vi "ScanBuilder.vi"(2 "Selected\nScan\nCorners":dbl[][](array[numeric])=[[211.0, 177.0, 58.0], [316.0, 213.0, 58.0]], 3 "ROI_Array 2":T3(array[cluster]) {"ROI begin channel" step=0.001; "ROI end channel" step=0.001; "Intensity" step=0.001; "Net Intensity" step=0.001; "Gauss Fit" step=0.001; "FWHM [keV]" step=0.001; "Center [keV]" step=0.001}) -> (0 "Do?":bool, 1 "ScanData":T4)   [LabVIEW 2015]
uses:
  Controls/String.ctl
  Controls/Number.ctl
panel:
  in  "PresetROI":u16(ring) items=["ca", "scat", "fe", "scat"]
  in  "Snake?":bool
  in  "Scan order:":u16(ring)=1 items=["X->Z->Y"=6, "Y->Z->X"=5, "Z->X->Y"=3, "Y->X->Z"=2, "Z->Y->X"=4, "X->Y->Z"=1]
  out "estimated duration":string caption="Estimated duration:"
  out "Output\nScan\nCorners":dbl[][](array[numeric])=[[211.0, 177.0, 58.0], [316.0, 213.0, 58.0]]
  in  "Accept":bool
  in  "Scan definition by:":enum32{"Step size", "Number of steps"}(radio)
  in  "Y steps":i32=1 min=1 step=1
  in  "X steps":i32=1 min=1 step=1
  out "total # of points":i32=1 min=0 step=1
  in  "step Y [mm]":dbl=1.0 min=0.0 step=0.1
  in  "step X [mm]":dbl=1.0 min=0.0 step=0.1
  in  "Cancel":bool
  in  "Preset type:":enum32{"Live time [s]", "Counts"}(radio)
  in  "ScanName:":string caption="Scan Name:"
  in  "PresetVal":dbl caption="Counts Preset"
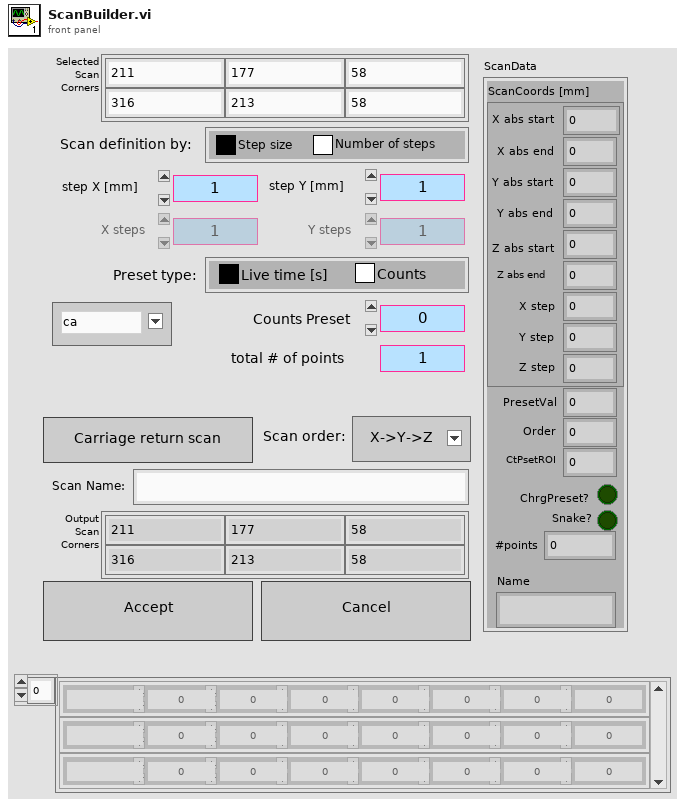
[diagram p1: front panel]
types:
  T1 = typedef "String.ctl" = string
  T2 = typedef "Number.ctl" = dbl
  T3 = cluster{"ROI name":T1, "ROI begin channel":T2, "ROI end channel":T2, "Intensity":T2, "Net Intensity":T2, "Gauss Fit":T2, "FWHM [keV]":T2, "Center [keV]":T2}[]
  T4 = cluster{"ScanCoords [mm]":cluster{"X abs start":dbl, "X abs end":dbl, "Y abs start":dbl, "Y abs end":dbl, "Z abs start":dbl, "Z abs end":dbl, "X step":dbl, "Y step":dbl, "Z step":dbl}, "PresetVal":dbl, "Order":u16, "Snake?":bool, "Name":string, "#points":i32, "ChrgPreset?":bool, "CtPsetROI":u16}
  T5 = cluster{"X abs start":dbl, "X abs end":dbl, "Y abs start":dbl, "Y abs end":dbl, "Z abs start":dbl, "Z abs end":dbl, "X step":dbl, "Y step":dbl, "Z step":dbl}
  T6 = enum8{"Enabled", "Disabled", "Disabled and Grayed Out"}
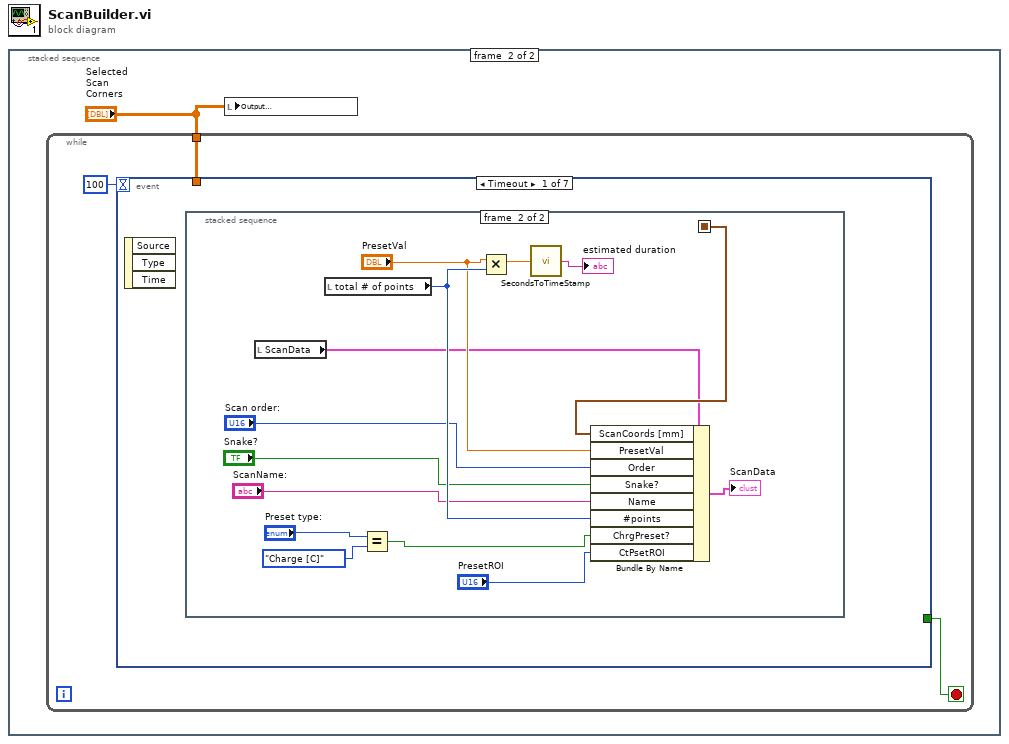
[diagram p0: block diagram]
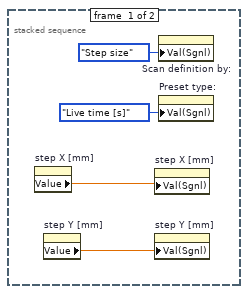
[diagram p2: hidden frame]
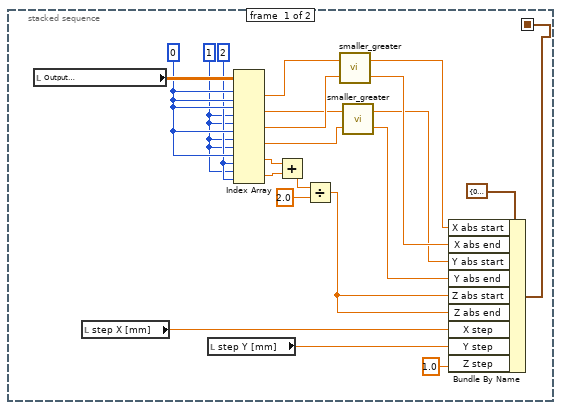
[diagram p3: hidden frame]
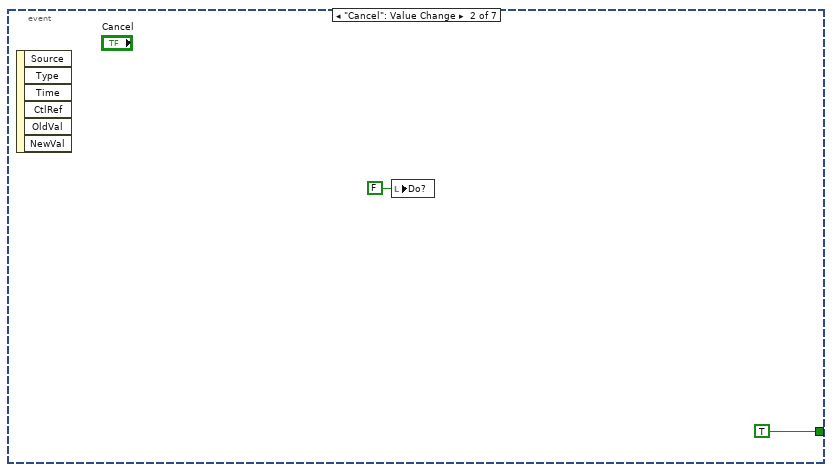
[diagram p4: hidden frame]
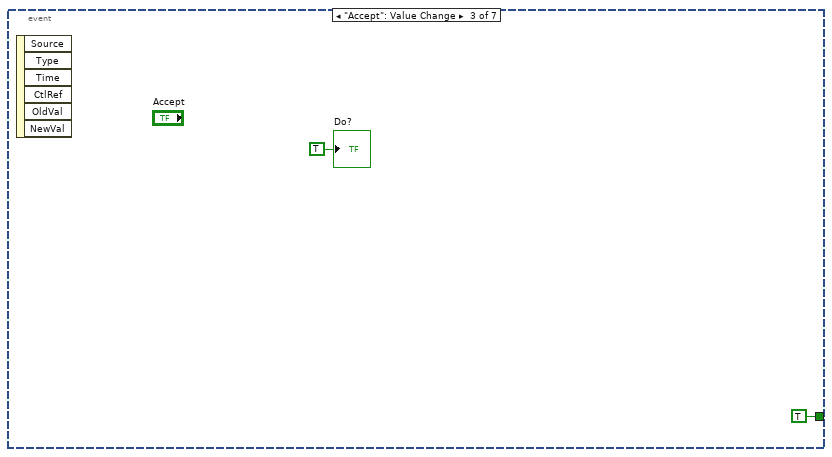
[diagram p5: hidden frame]
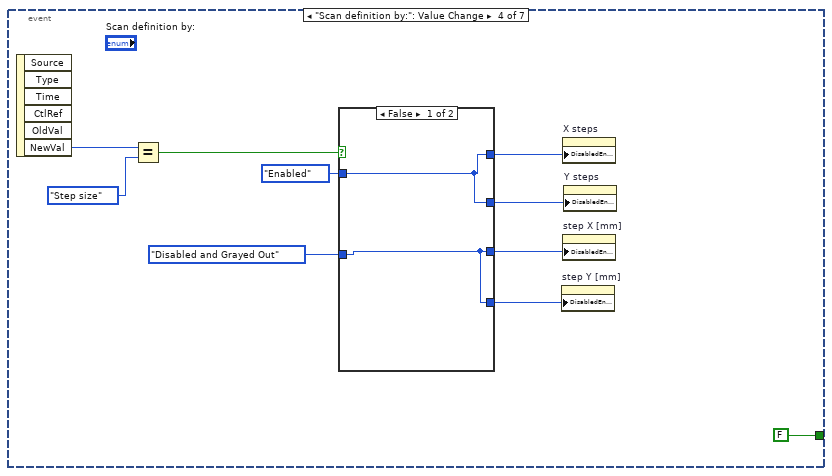
[diagram p6: hidden frame]
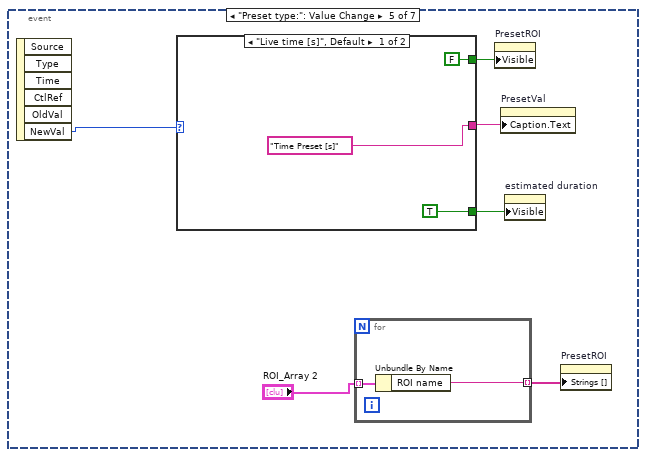
[diagram p8: hidden frame]
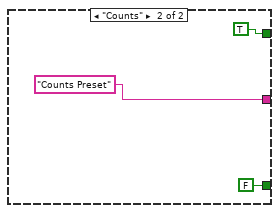
[diagram p9: hidden frame]
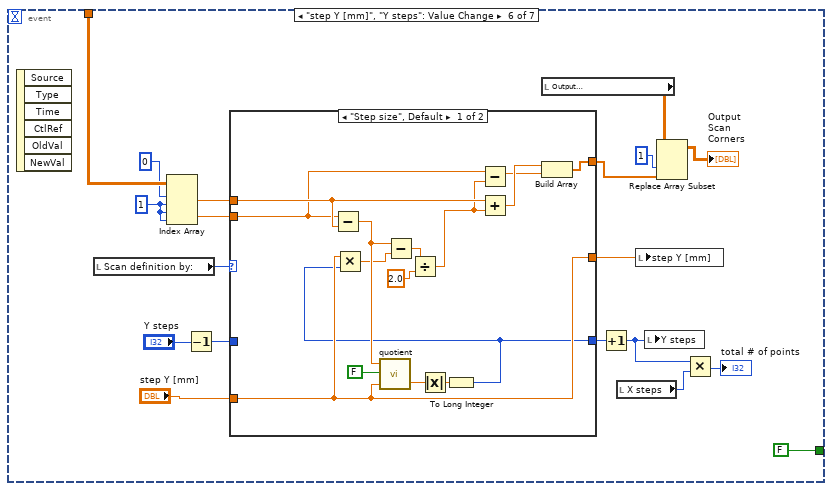
[diagram p10: hidden frame]
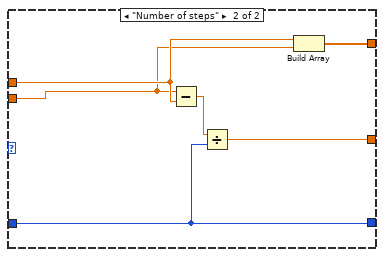
[diagram p11: hidden frame]
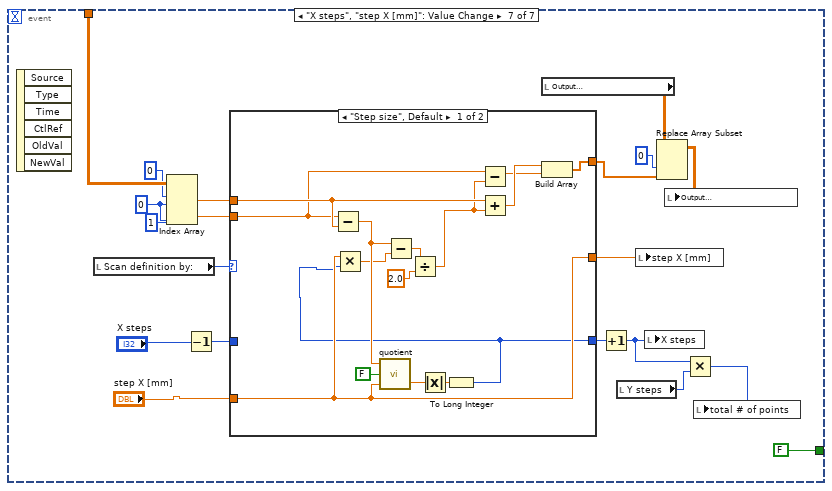
[diagram p12: hidden frame]
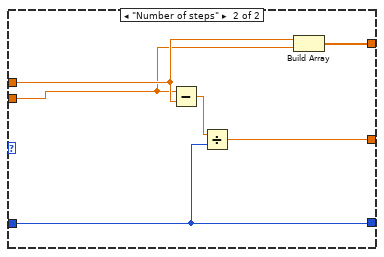
[diagram p13: hidden frame]
diagram:
  n1 = stacked-sequence {
    frame #0 {
      n2 = property on="step X [mm]" class="DigNum (strict)"() -> ("Value"=w3:dbl)  [unwired: 2 in, 2 out]
      n3 = property on="step Y [mm]" class="DigNum (strict)"() -> ("Value"=w2:dbl)  [unwired: 2 in, 2 out]
      n4 = property on="step X [mm]" class="DigNum (strict)"("Val(Sgnl)"=w3) -> ()  [unwired: 2 in, 2 out]
      n5 = property on="step Y [mm]" class="DigNum (strict)"("Val(Sgnl)"=w2) -> ()  [unwired: 2 in, 2 out]
      n6 = property on="Scan definition by:" class="RadioBtnsControl (strict)"("Val(Sgnl)"=enum32{"Step size", "Number of steps"}."Step size" ("Value (Signaling)")) -> ()  [unwired: 2 in, 2 out]
      n7 = property on="Preset type:" class="RadioBtnsControl (strict)"("Val(Sgnl)"=enum32{"Live time [s]", "Counts"}."Live time [s]" ("Value (Signaling)")) -> ()  [unwired: 2 in, 2 out]
    }
    frame #1 {
      n8 = while {
        tunnel: "Selected\nScan\nCorners" -> [w6]
        stop <- w7 stop-if-true
        n9 = event shown="[0] Timeout" {
          selector: _ -> [_ _ _ _ _ _ _]
          dyn-events: _ -> [_ _ _ _ _ _ _]
          timeout: 100 -> [_ _ _ _ _ _ _]
          tunnel: [_ TRUE TRUE FALSE _ FALSE FALSE] -> w7
          tunnel: w6 -> [_ _ _ _ _ w94 w135]
          event Timeout {
            n10 = event-data() -> ()  [unwired: 1 in, 3 out]
            n11 = stacked-sequence {
              seq-local: [w18 _] -> [_ w40]
              frame #0 {
                w27 = 2 ("disabled index (col)")
                w26 = 1 ("disabled index (col)")
                w28 = 0 ("index (row)")
                n12 = local read "Output\nScan\nCorners"() -> (w29:dbl[][])
                n13 = local read "step X [mm]"() -> (w25:dbl)
                n14 = local read "step Y [mm]"() -> (w24:dbl)
                n15 = Index Array(array=w29, index (row) #1=w28, index (col) #1=w28, index (row) #2=w28, index (col) #2=w26, index (row) #3=w26, index (col) #3=w28, index (row) #4=w26, index (col) #4=w26, index (row) #5=w28, index (col) #5=w27, index (row) #6=w26, index (col) #6=w27) -> (element #1=w13:dbl, element #2=w10:dbl, element #3=w14:dbl, element #4=w9:dbl, element #5=w23:dbl, element #6=w22:dbl)
                n16 = Add(x=w23, y=w22) -> (x+y=w21:dbl)
                n17 = Divide(x=w21, y=2.0) -> (x/y=w19:dbl)
                n18 = call "smaller_greater.vi"("input 2"=w14, "input 1"=w13) -> ("greater"=w15:dbl, "smaller"=w16:dbl)
                n19 = call "smaller_greater.vi"("input 2"=w9, "input 1"=w10) -> ("greater"=w11:dbl, "smaller"=w12:dbl)
                n20 = Bundle By Name(cluster=T5 {"X abs start"=0.0, "X abs end"=0.0, "Y abs start"=0.0, "Y abs end"=0.0, "Z abs start"=0.0, "Z abs end"=0.0, "X step"=0.0, "Y step"=0.0, "Z step"=0.0} ("ScanCoords [mm] 2"), "X abs start"=w16, "X abs end"=w15, "Y abs start"=w12, "Y abs end"=w11, "Z abs start"=w19, "Z abs end"=w19, "X step"=w25, "Y step"=w24, "Z step"=1.0) -> (w18:T5)
              }
              frame #1 {
                n21 = local read "ScanData"() -> (w39:T4)
                n22 = local read "total # of points"() -> (w42:i32)
                n23 = Equal?(x="Preset type:", y=enum32{"Live time [s]", "Charge [C]"}."Charge [C]" ("Preset type:")) -> (x = y?=w32:bool)
                n24 = Multiply(x="PresetVal", y=w42) -> (x*y=w43:dbl)
                n25 = call "SecondsToTimeStamp.vi"("Time [s]"=w43) -> ("TimeStamp"=→"estimated duration":string)
                n26 = Bundle By Name(cluster=w39, "ScanCoords [mm]"=w40, "PresetVal"="PresetVal", "Order"="Scan order:", "Snake?"="Snake?", "Name"="ScanName:", "#points"=w42, "ChrgPreset?"=w32, "CtPsetROI"="PresetROI") -> (→"ScanData":T4)
              }
            }
          }
          event "Cancel": Value Change {
            n27 = event-data() -> ()  [unwired: 1 in, 6 out]
            n28 = local write "Do?"(FALSE ("Do?")) -> ()
          }
          event "Accept": Value Change {
            n29 = event-data() -> ()  [unwired: 1 in, 6 out]
            "Do?" <- TRUE ("Do?")
          }
          event "Scan definition by:": Value Change {
            n30 = event-data() -> ("NewVal"=w58:enum32{"Step size", "Number of steps"})  [unwired: 1 in, 5 out]
            n31 = Equal?(x=w58, y=enum32{"Step size", "Number of steps"}."Step size" ("Scan definition by:")) -> (x = y?=w56:bool)
            n32 = case shown="False" w56 {
              tunnel: [w60 w61] -> w55
              tunnel: [w60 w61] -> w54
              tunnel: [w59 w62] -> w53
              tunnel: [w59 w62] -> w52
              tunnel: T6."Enabled" ("Disabled") -> [w60 w62]
              tunnel: T6."Disabled and Grayed Out" ("Disabled") -> [w59 w61]
              frame False {
              }
              frame True {
              }
            }
            n33 = property on="step Y [mm]" class="DigNum (strict)"("DisabledEnum"=w52) -> ()  [unwired: 2 in, 2 out]
            n34 = property on="X steps" class="DigNum (strict)"("DisabledEnum"=w55) -> ()  [unwired: 2 in, 2 out]
            n35 = property on="step X [mm]" class="DigNum (strict)"("DisabledEnum"=w53) -> ()  [unwired: 2 in, 2 out]
            n36 = property on="Y steps" class="DigNum (strict)"("DisabledEnum"=w54) -> ()  [unwired: 2 in, 2 out]
          }
          event "Preset type:": Value Change {
            n37 = event-data() -> ("NewVal"=w68:enum32{"Live time [s]", "Counts"})  [unwired: 1 in, 5 out]
            n38 = case shown="\"Live time [s]\", Default" w68 {
              tunnel: ["Time Preset [s]" ("Caption.Text") "Counts Preset" ("Caption.Text")] -> w67
              tunnel: [TRUE FALSE] -> w66
              tunnel: [FALSE TRUE] -> w63
              frame "Live time [s]", Default {
              }
              frame "Counts" {
              }
            }
            n39 = for {
              tunnel: "ROI_Array 2" -> [w70] mode=indexing
              tunnel: [w69] -> w64 mode=indexing
              n40 = Unbundle By Name(w70) -> ("ROI name"=w69:T1)
            }
            n41 = property on="PresetROI" class="Ring (strict)"("Visible"=w63) -> ()  [unwired: 2 in, 2 out]
            n42 = property on="PresetVal" class="DigNum (strict)"("Caption.Text"=w67) -> ()  [unwired: 2 in, 2 out]
            n43 = property on="estimated duration" class="Str"("Visible"=w66) -> ()  [unwired: 2 in, 2 out]
            n44 = property on="PresetROI" class="Ring (strict)"("Strings []"=w64) -> ()  [unwired: 2 in, 2 out]
          }
          event "step Y [mm]", "Y steps": Value Change {
            w93 = 1 ("disabled index (col)")
            n45 = event-data() -> ()  [unwired: 1 in, 6 out]
            n46 = local read "Scan definition by:"() -> (w91:enum32{"Step size", "Number of steps"})
            n47 = Index Array(array=w94, index (row) #1=0 ("disabled index (row)"), index (col) #1=w93, index (row) #2=w93, index (col) #2=w93) -> (element #1=w90:dbl, element #2=w89:dbl)
            n48 = Decrement(x="Y steps") -> (x-1=w86:i32)
            n49 = case shown="\"Step size\", Default" w91 {
              tunnel: w90 -> [w103 w113]
              tunnel: w89 -> [w102 w112]
              tunnel: [w108 w115] -> w88
              tunnel: w86 -> [_ w114]
              tunnel: [w97 w114] -> w85
              tunnel: "step Y [mm]" -> [w108 _]
              tunnel: [w98 w111] -> w79
              frame "Step size", Default {
                n50 = Subtract(x=w102, y=w103) -> (x-y=w107:dbl)
                n51 = call "quotient.vi"("Y"=w108, "Nearest?"=FALSE, "X"=w107) -> ("s? t:f"=w109:dbl)  [unwired: 1 out]
                n52 = Absolute Value(x=w109) -> (abs(x)=w110:dbl)
                n53 = To Long Integer(number=w110) -> (32bit integer=w97:i32)
                n54 = Multiply(x=w108, y=w97) -> (x*y=w106:dbl)
                n55 = Subtract(x=w107, y=w106) -> (x-y=w105:dbl)
                n56 = Divide(x=w105, y=2.0) -> (x/y=w101:dbl)
                n57 = Subtract(x=w102, y=w101) -> (x-y=w99:dbl)
                n58 = Add(x=w103, y=w101) -> (x+y=w100:dbl)
                n59 = Build Array(w100, w99) -> (w98:dbl[])
              }
              frame "Number of steps" {
                n60 = Subtract(x=w112, y=w113) -> (x-y=w116:dbl)
                n61 = Divide(x=w116, y=w114) -> (x/y=w115:dbl)
                n62 = Build Array(w113, w112) -> (w111:dbl[])
              }
            }
            n63 = local read "Output\nScan\nCorners"() -> (w80:dbl[][])
            n64 = Increment(x=w85) -> (x+1=w84:i32)
            n65 = local read "X steps"() -> (w83:i32)
            n66 = local write "step Y [mm]"(w88) -> ()
            n67 = local write "Y steps"(w84) -> ()
            n68 = Replace Array Subset(array=w80, new element=w79, index (col)=1 ("disabled index (col)")) -> (→"Output\nScan\nCorners":dbl[][])  [unwired: 1 in]
            n69 = Multiply(x=w84, y=w83) -> (x*y=→"total # of points":i32)
          }
          event "X steps", "step X [mm]": Value Change {
            w134 = 0 ("disabled index (col)")
            n70 = event-data() -> ()  [unwired: 1 in, 6 out]
            n71 = local read "Scan definition by:"() -> (w132:enum32{"Step size", "Number of steps"})
            n72 = Index Array(array=w135, index (row) #1=0 ("disabled index (row)"), index (col) #1=w134, index (row) #2=1 ("disabled index (row)"), index (col) #2=w134) -> (element #1=w131:dbl, element #2=w130:dbl)
            n73 = Decrement(x="X steps") -> (x-1=w128:i32)
            n74 = case shown="\"Step size\", Default" w132 {
              tunnel: w131 -> [w144 w154]
              tunnel: w130 -> [w143 w153]
              tunnel: [w149 w156] -> w129
              tunnel: w128 -> [_ w155]
              tunnel: [w138 w155] -> w127
              tunnel: "step X [mm]" -> [w149 _]
              tunnel: [w139 w152] -> w123
              frame "Step size", Default {
                n75 = Subtract(x=w143, y=w144) -> (x-y=w148:dbl)
                n76 = call "quotient.vi"("Y"=w149, "Nearest?"=FALSE, "X"=w148) -> ("s? t:f"=w150:dbl)  [unwired: 1 out]
                n77 = Absolute Value(x=w150) -> (abs(x)=w151:dbl)
                n78 = To Long Integer(number=w151) -> (32bit integer=w138:i32)
                n79 = Multiply(x=w149, y=w138) -> (x*y=w147:dbl)
                n80 = Subtract(x=w148, y=w147) -> (x-y=w146:dbl)
                n81 = Divide(x=w146, y=2.0) -> (x/y=w142:dbl)
                n82 = Subtract(x=w143, y=w142) -> (x-y=w140:dbl)
                n83 = Add(x=w144, y=w142) -> (x+y=w141:dbl)
                n84 = Build Array(w141, w140) -> (w139:dbl[])
              }
              frame "Number of steps" {
                n85 = Subtract(x=w153, y=w154) -> (x-y=w157:dbl)
                n86 = Divide(x=w157, y=w155) -> (x/y=w156:dbl)
                n87 = Build Array(w154, w153) -> (w152:dbl[])
              }
            }
            n88 = local read "Output\nScan\nCorners"() -> (w124:dbl[][])
            n89 = Increment(x=w127) -> (x+1=w126:i32)
            n90 = local read "Y steps"() -> (w125:i32)
            n91 = local write "step X [mm]"(w129) -> ()
            n92 = local write "X steps"(w126) -> ()
            n93 = Replace Array Subset(array=w124, new element=w123, index (col)=0 ("disabled index (col)")) -> (w119:dbl[][])  [unwired: 1 in]
            n94 = local write "Output\nScan\nCorners"(w119) -> ()
            n95 = Multiply(x=w126, y=w125) -> (x*y=w118:i32)
            n96 = local write "total # of points"(w118) -> ()
          }
        }
      }
      n97 = local write "Output\nScan\nCorners"("Selected\nScan\nCorners") -> ()
    }
  }
